vi "launch background process.vi"(8 "error in":errorcluster, 10 "data allocations":T1, 11 "asynchronous execution module runtime In":refnum<class "asynchronous execution module runtime.lvclass">) -> (0 "error out":errorcluster, 3 "asynchronous execution module runtime Out":refnum<class "asynchronous execution module runtime.lvclass">)   [LabVIEW 2013, in "asynchronous execution module runtime.lvclass"]
uses:
  asynchronous execution module runtime.lvclass
  <vilib>/NI/Tag Bus Module Framework/channel/data tables.ctl
  <vilib>/NI/Tag Bus/dictionary/data dictionary.lvclass
  <vilib>/NI/Tag Bus/dictionary table pair.ctl
  <vilib>/NI/Tag Bus/table/data table.ctl
  asynchronous execution module runtime.lvclass/asynchronous execution module runtime.ctl
  <vilib>/NI/Tag Bus/table/data table.lvlib
  <vilib>/NI/Tag Bus/tag bus.lvlib
  <vilib>/NI/Tag Bus Module Framework/channel/TBM channel.lvclass
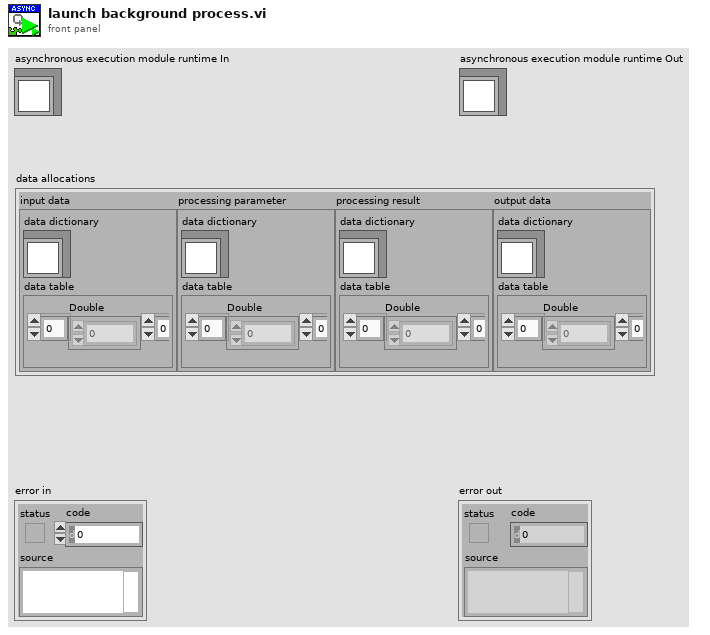
[diagram p1: front panel]
types:
  T1 = typedef "TBM channel.lvclass/data tables.ctl" = cluster{"input data":T2, "processing parameter":T2, "processing result":T2, "output data":T2}
  T2 = typedef "tag bus.lvlib/dictionary table pair.ctl" = cluster{"data dictionary":refnum<class "data dictionary.lvclass">, "data table":T3}
  T3 = typedef "tag bus.lvlib/data table.lvlib/data table.ctl" = cluster{"Double":dbl[], "Single":sgl[], "I64":i64[], "I32":i32[], "I16":i16[], "I8":i8[], "U64":u64[], "U32":u32[], "U16":u16[], "U8":u8[], "Boolean":bool[], "String":string[], "Array of Double":cluster{"DBL Array":dbl[]}[], "Array of Single":cluster{"SGL Array":sgl[]}[], "Array of I64":cluster{"I64 Array":i64[]}[], "Array of I32":cluster{"I32 Array":i32[]}[], "Array of I16":cluster{"I16 Array":i16[]}[], "Array of I8":cluster{"I8 Array":i8[]}[], "Array of U64":cluster{"U64 Array":u64[]}[], "Array of U32":cluster{"U32 Array":u32[]}[], "Array of U16":cluster{"U16 Array":u16[]}[], "Array of U8":cluster{"U8 Array":u8[]}[], "Array of Boolean":cluster{"Boolean Array":bool[]}[], "Array of String":cluster{"String Array":string[]}[]}
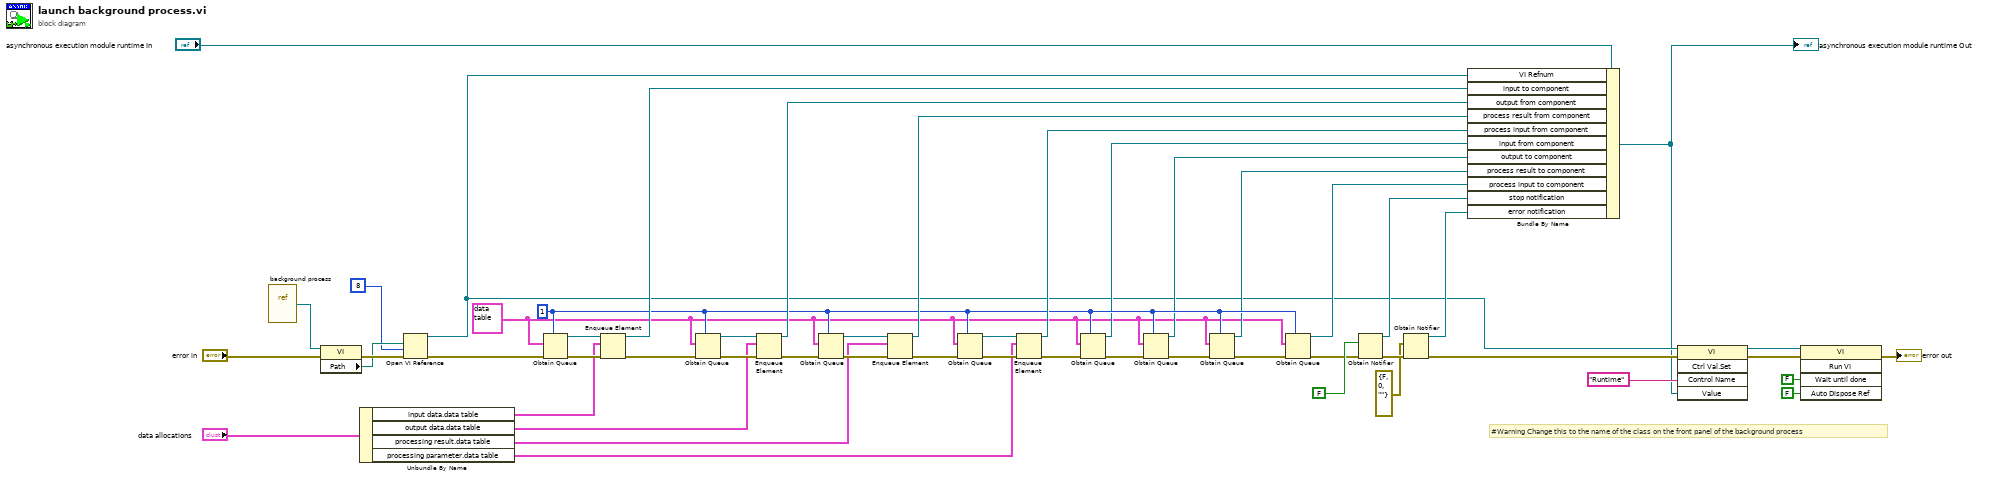
[diagram p0: block diagram]
diagram:
  w4 = T3 {"Double"=[], "Single"=[], "I64"=[], "I32"=[], "I16"=[], "I8"=[], "U64"=[], "U32"=[], "U16"=[], "U8"=[], "Boolean"=[], "String"=[], "Array of Double"=[], "Array of Single"=[], "Array of I64"=[], "Array of I32"=[], "Array of I16"=[], "Array of I8"=[], "Array of U64"=[], "Array of U32"=[], "Array of U16"=[], "Array of U8"=[], "Array of Boolean"=[], "Array of String"=[]} ("input data")
  w17 = 1 ("max queue size (-1, unlimited)")
  # "#Warning Change this to the name of the class on the front panel of the background process"
  n1 = vi-ref "background process.vi"() -> (w49:refnum<vi>)
  n2 = property class="VI"(reference=w49, error in="error in") -> (error out=w50:errorcluster, "Path"=w48:path)  [unwired: 1 out]
  n3 = Unbundle By Name("data allocations") -> ("input data.data table"=w26:T3, "output data.data table"=w25:T3, "processing result.data table"=w24:T3, "processing parameter.data table"=w23:T3)
  n4 = Open VI Reference(vi path=w48, options=8, error in (no error)=w50) -> (vi reference=w11:refnum<vi>, error out=w47:errorcluster)  [unwired: 3 in]
  n5 = Obtain Queue(max queue size (-1, unlimited)=w17, element data type=w4, error in (no error)=w47) -> (queue out=w36:refnum<queue>, error out=w46:errorcluster)  [unwired: 2 in, 1 out]
  n6 = Enqueue Element(queue=w36, element=w26, error in (no error)=w46) -> (queue out=w35:refnum<queue>, error out=w37:errorcluster)  [unwired: 1 in, 1 out]
  n7 = Obtain Queue(max queue size (-1, unlimited)=w17, element data type=w4, error in (no error)=w37) -> (queue out=w30:refnum<queue>, error out=w45:errorcluster)  [unwired: 2 in, 1 out]
  n8 = Enqueue Element(queue=w30, element=w25, error in (no error)=w45) -> (queue out=w29:refnum<queue>, error out=w31:errorcluster)  [unwired: 1 in, 1 out]
  n9 = Obtain Queue(max queue size (-1, unlimited)=w17, element data type=w4, error in (no error)=w31) -> (queue out=w33:refnum<queue>, error out=w44:errorcluster)  [unwired: 2 in, 1 out]
  n10 = Enqueue Element(queue=w33, element=w24, error in (no error)=w44) -> (queue out=w32:refnum<queue>, error out=w34:errorcluster)  [unwired: 1 in, 1 out]
  n11 = Obtain Queue(max queue size (-1, unlimited)=w17, element data type=w4, error in (no error)=w34) -> (queue out=w28:refnum<queue>, error out=w43:errorcluster)  [unwired: 2 in, 1 out]
  n12 = Enqueue Element(queue=w28, element=w23, error in (no error)=w43) -> (queue out=w27:refnum<queue>, error out=w18:errorcluster)  [unwired: 1 in, 1 out]
  n13 = Obtain Queue(max queue size (-1, unlimited)=w17, element data type=w4, error in (no error)=w18) -> (queue out=w13:refnum<queue>, error out=w19:errorcluster)  [unwired: 2 in, 1 out]
  n14 = Obtain Queue(max queue size (-1, unlimited)=w17, element data type=w4, error in (no error)=w19) -> (queue out=w14:refnum<queue>, error out=w20:errorcluster)  [unwired: 2 in, 1 out]
  n15 = Obtain Queue(max queue size (-1, unlimited)=w17, element data type=w4, error in (no error)=w20) -> (queue out=w15:refnum<queue>, error out=w21:errorcluster)  [unwired: 2 in, 1 out]
  n16 = Obtain Queue(max queue size (-1, unlimited)=w17, element data type=w4, error in (no error)=w21) -> (queue out=w16:refnum<queue>, error out=w22:errorcluster)  [unwired: 2 in, 1 out]
  n17 = Obtain Notifier(notification data type=FALSE, error in (no error)=w22) -> (notifier out=w38:refnum<notifier>, error out=w42:errorcluster)  [unwired: 2 in, 1 out]
  n18 = Obtain Notifier(notification data type=errorcluster {"status"=FALSE, "code"=0, "source"=""} ("error constant"), error in (no error)=w42) -> (notifier out=w41:refnum<notifier>, error out=w12:errorcluster)  [unwired: 2 in, 1 out]
  n19 = Bundle By Name(cluster="asynchronous execution module runtime In", "VI Refnum"=w11, "input to component"=w35, "output from component"=w29, "process result from component"=w32, "process input from component"=w27, "input from component"=w13, "output to component"=w14, "process result to component"=w15, "process input to component"=w16, "stop notification"=w38, "error notification"=w41) -> (w1:refnum<class "asynchronous execution module runtime.lvclass">)
  "asynchronous execution module runtime Out" <- w1
  n20 = invoke class="VI" method="Ctrl Val.Set"(reference=w11, error in=w12, "Control Name"="Runtime", "Value"=w1) -> (reference out=w9:refnum<vi>, error out=w8:errorcluster)  [unwired: 1 in, 3 out]
  n21 = invoke class="VI" method="Run VI"(reference=w9, error in=w8, "Wait until done"=FALSE ("Wait Until Done"), "Auto Dispose Ref"=FALSE ("Auto Dispose Reference")) -> (error out=→"error out":errorcluster)  [unwired: 1 in, 4 out]
